vi "Read signal settings.vi"(1 "base path":path) -> (14 "channel name(s) in (Untitled)":string[](array[string])=["Encoder signal", "Photo-diode", "Distance (cm)", "Position in Unity", "Valve open", "Lick signal", "Analog lick signal", "VR context", "VR gain"], 15 "Save":bool[](array[boolean]), 16 "channel name(s) in (Untitled) 2":string[](array[string])=["Frame signal", "Frame signal 2", "EyeCam frame signal", "Analog input 3"], 17 "Save 2":bool[](array[boolean]), 18 "channel name(s) in (Untitled) 3":string[](array[string])=["Photo stimulus signal", "Masking light signal", "Stimulus protocol", "Analog input 5"], 19 "Save 3":bool[](array[boolean]))   [LabVIEW 2017]
uses:
  <vilib>/Utility/file.llb/Read Delimited Spreadsheet (string).vi
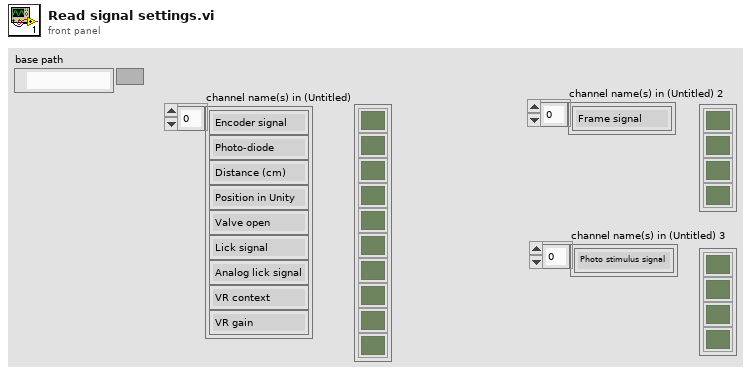
[diagram p1: front panel]
types:
  T1 = enum16{"open", "replace", "create", "open or create", "replace or create", "replace or create with confirmation"}
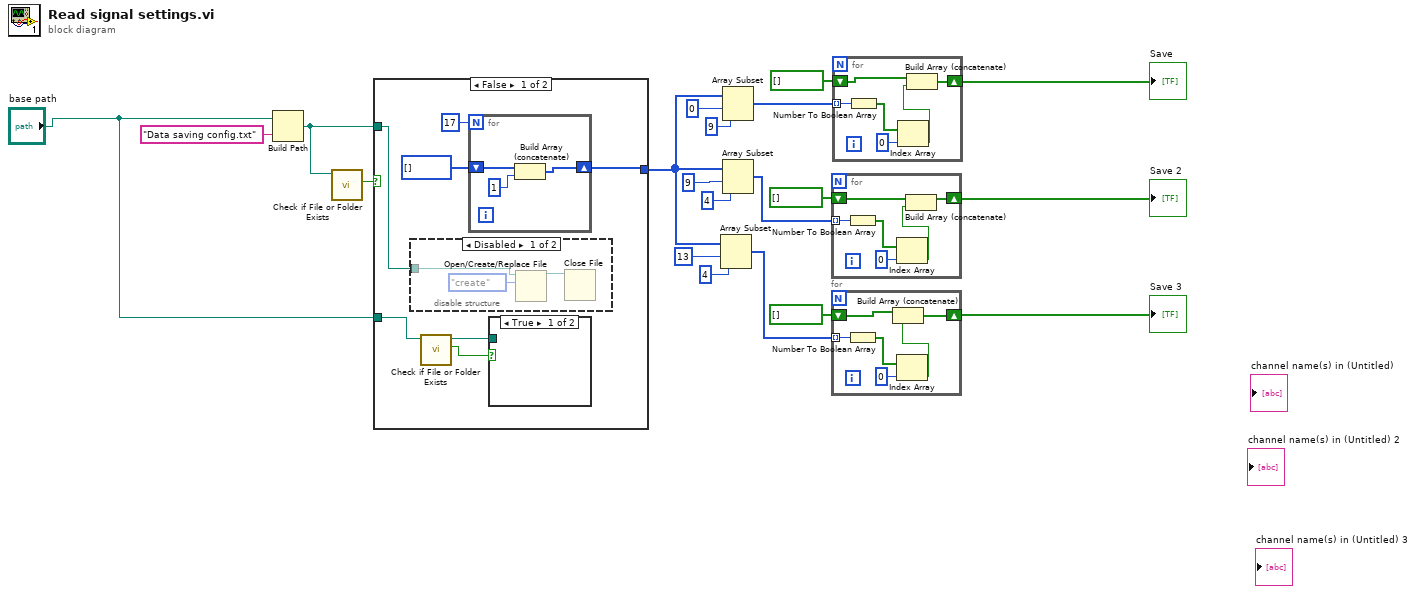
[diagram p0: block diagram]
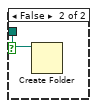
[diagram p2: hidden frame]
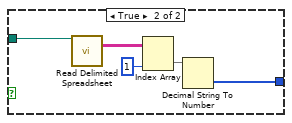
[diagram p4: hidden frame]
diagram:
  n1 = Build Path(base path="base path", name or relative path="Data saving config.txt") -> (appended path=w6:path)
  n2 = call <vilib>:"Check if File or Folder Exists.vi"("path"=w6) -> ("file or folder exists?"=w5:bool)  [unwired: 8 in, 2 out]
  n3 = case shown="False" w5 {
    tunnel: [w27 w36] -> w13
    tunnel: w6 -> [w24 w35]
    tunnel: "base path" -> [w23 _]
    frame False {
      n4 = disable-structure shown="Disabled" {
        disable-tunnel: w24 -> [w29 _]
        frame Disabled {
          n5 = Open/Create/Replace File(file path (use dialog)=w29, operation (0:open)=T1."create") -> (refnum out=w30:refnum<file>)  [unwired: 4 in, 2 out]
          n6 = Close File(refnum=w30) -> ()  [unwired: 1 in, 2 out]
        }
        frame Enabled {
        }
      }
      n7 = call <vilib>:"Check if File or Folder Exists.vi"("path"=w23) -> ("file or folder exists?"=w21:bool, "dup path"=w22:path)  [unwired: 8 in, 1 out]
      n8 = for {
        N: 17 -> [_]
        shift-right: [w33] -> w27
        shift-left: i32[] [] -> [w34]
        n9 = Build Array (concatenate)(w34, 1 ("index")) -> (w33:i32[])
      }
      n10 = case shown="True" w21 {
        tunnel: w22 -> [_ w28]
        frame True {
        }
        frame False {
          n11 = Create Folder(path (use dialog)=w28) -> ()  [unwired: 2 in, 3 out]
        }
      }
    }
    frame True {
      n12 = call-poly <vilib>:"Read Delimited Spreadsheet.vi"("file path (dialog if empty)"=w35) -> ("all rows"=w39:string[][])  [unwired: 9 in, 5 out]
      n13 = Index Array(array=w39, index (col)=1 ("disabled index (col)")) -> (element=w37:string[])  [unwired: 1 in]
      n14 = Decimal String To Number(string=w37) -> (number=w36:i32[])  [unwired: 2 in, 1 out]
    }
  }
  n15 = Array Subset(array=w13, index=13, length=4) -> (w7:i32[])
  n16 = Array Subset(array=w13, index=0, length=9) -> (w12:i32[])
  n17 = Array Subset(array=w13, index=9, length=4) -> (w8:i32[])
  n18 = for {
    tunnel: w8 -> [w45] mode=indexing
    shift-right: [w41] -> w3
    shift-left: bool[] [] -> [w40]
    n19 = Number To Boolean Array(number=w45) -> (Boolean array=w43:bool[])
    n20 = Index Array(array=w43, index=0) -> (element=w44:bool)
    n21 = Build Array (concatenate)(w40, w44) -> (w41:bool[])
  }
  "Save 2" <- w3
  n22 = for {
    tunnel: w7 -> [w51] mode=indexing
    shift-right: [w47] -> w2
    shift-left: bool[] [] -> [w46]
    n23 = Number To Boolean Array(number=w51) -> (Boolean array=w49:bool[])
    n24 = Index Array(array=w49, index=0) -> (element=w50:bool)
    n25 = Build Array (concatenate)(w46, w50) -> (w47:bool[])
  }
  "Save 3" <- w2
  n26 = for {
    tunnel: w12 -> [w57] mode=indexing
    shift-right: [w53] -> w4
    shift-left: bool[] [] -> [w52]
    n27 = Number To Boolean Array(number=w57) -> (Boolean array=w55:bool[])
    n28 = Index Array(array=w55, index=0) -> (element=w56:bool)
    n29 = Build Array (concatenate)(w52, w56) -> (w53:bool[])
  }
  "Save" <- w4
